vi "Lyapunov Equations.vi"   [LabVIEW 2017, in "NI_AALPro.lvlib"]
doc: "Solves the Lyapunov matrix equation. The data types you wire to the <B>A</B> and <B>B</B> inputs determine the polymorphic instance to use."
uses:
  <vilib>/Analysis/NI_AALPro.lvlib
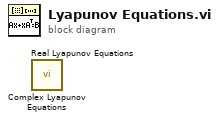
[diagram p0: block diagram]
diagram:
  n1 = call <vilib>:"Complex Lyapunov Equations.vi"() -> ()  [unwired: 9 in, 3 out]
  n2 = call <vilib>:"Real Lyapunov Equations.vi"() -> ()  [unwired: 9 in, 3 out]
